vi "Build Histogram Node Paths.vi"(9 "Upper Bounds":dbl[](array[numeric]), 10 "Lower Bounds":dbl[](array[numeric]), 11 "Selected Item":string) -> (3 "Node Paths":string[](array[string]))   [LabVIEW 2012]
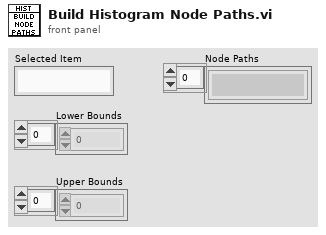
[diagram p1: front panel]
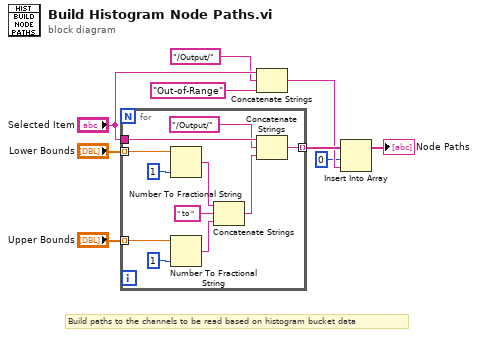
[diagram p0: block diagram]
diagram:
  # "Build paths to the channels to be read based on histogram bucket data"
  n1 = for {
    tunnel: "Lower Bounds" -> [w19] mode=indexing
    tunnel: "Upper Bounds" -> [w20] mode=indexing
    tunnel: "Selected Item" -> [w13]
    tunnel: [w10] -> w7 mode=indexing
    n2 = Number To Fractional String(number=w19, precision (6)=i16 1) -> (F-format string=w18:string)  [unwired: 2 in]
    n3 = Number To Fractional String(number=w20, precision (6)=i16 1) -> (F-format string=w17:string)  [unwired: 2 in]
    n4 = Concatenate Strings(w18, " to " ("string"), w17) -> (w11:string)
    n5 = Concatenate Strings(w13, "/Output/" ("string"), w11) -> (w10:string)
  }
  n6 = Concatenate Strings("Selected Item", "/Output/" ("string"), "Out-of-Range" ("string")) -> (w3:string)
  n7 = Insert Into Array(array=w7, index=0, new element=w3) -> (→"Node Paths":string[])
